vi "App Top Level Tasks.vi"(8 "error in (no error)":errorcluster, 11 "DemoApp in":refnum<class "DemoApp.lvclass">) -> (0 "error out":errorcluster, 2 "Top Level Tasks":refnum<class "Task.lvclass">[](array[class]))   [LabVIEW 2020, in "VolatusDemo.lvlib" / "DemoApp.lvclass"]
uses:
  DemoApp.lvclass
  Volatus/Task/Task.lvclass
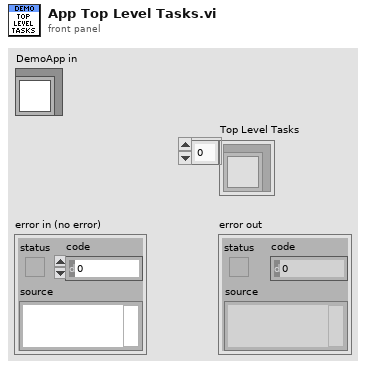
[diagram p1: front panel]
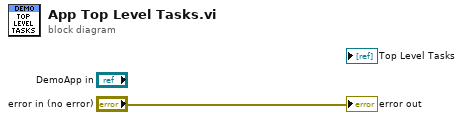
[diagram p0: block diagram]
diagram:
  "error out" <- "error in (no error)"
